vi "checkSetCurrent.vi"(8 "error in (no error)":errorcluster) -> (0 "DS read error":errorcluster)   [LabVIEW 2013]
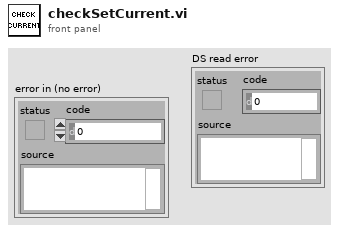
[diagram p1: front panel]
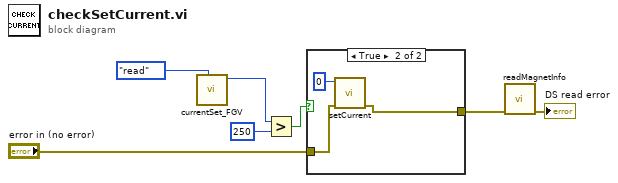
[diagram p0: block diagram]
diagram:
  n1 = call "currentSet_FGV.vi"("Enum"=enum16{"set", "read"}."read") -> ("curent set out"=w3:u16)  [unwired: 10 in]
  n2 = Greater?(x=w3, y=u16 250) -> (0:w5:bool)
  n3 = case shown="True" w5 {
    tunnel: [w8 w10] -> w6
    tunnel: "error in (no error)" -> [w8 w9]
    frame False {
    }
    frame True {
      n4 = call "setCurrent.vi"("error in (no error)"=w9, "curent set"=u16 0) -> ("error out"=w10:errorcluster)  [unwired: 9 in]
    }
  }
  n5 = call "readMagnetInfo.vi"("error in (no error)"=w6) -> ("DS read error"=→"DS read error":errorcluster)  [unwired: 9 in, 1 out]
